vi "Initialise camera.vi"(8 "error in (no error) 2":errorcluster, 10 "Camera configuration":T4={"Temperature"=-70.0, "Exposure (sec)"=0.01, "EMGain"=3500.0, "ClearMode"=1.0, "ReadoutMode"=2.0, "ADC Gain"=-1} {"ADC Gain" items=["Use current ADC"=-1, "Use the fastest ADC"=-2, "Use the slowest ADC"=-3]; "ReadoutMode" items=["Normal readout"=1.0, "Frame transfer readout"=2.0, "MPP readout"=3.0, "Frame transfer MPP"=4.0, "Alternate timing for normal readout"=5.0, "Alternate timing for frame transfer"=6.0, "Alternate timing for MPP"=7.0, "Alternate timing for frame transfer MPP"=8.0, "Interline"=9.0]; "ClearMode" items=["Clear never"=1.0, "Clear pre-exposure"=2.0, "Clear pre-sequence"=3.0, "Clear post-sequence"=4.0, "Clear pre- and post-sequence"=5.0, "Clear pre-exposure and post-sequence"=6.0]; "EMGain" format="%.2f"; "Exposure (sec)" format="%.3f"; "Temperature" format="%.2f"}, 11 "Acqusition Info":T8={"Number of Images"=1000, "Image type"=6, "Acquire / Focus Flag"=1} {"Image type" items=["8 bit unsigned"=1, "16 bit unsigned"=2, "8 bit signed"=6, "16 bit signed"=7, "32 bit signed"=3, "32 bit floating"=4, "64 bit floating"=5, "32 bit unsigned"=8]}) -> (0 "error out":errorcluster, 2 "Camera Info":T6, 3 "Imafe Info":T5)   [LabVIEW 2012, in "DAQCascade512.lvclass"]
uses:
  DAQCascade512.lvclass
  OLD_apparatus_VI/VI/Image_type.ctl
  OLD_apparatus_VI/VI/Clearing_mode.ctl
  OLD_apparatus_VI/VI/Readout_mode.ctl
  OLD_apparatus_VI/VI/ADC_gain.ctl
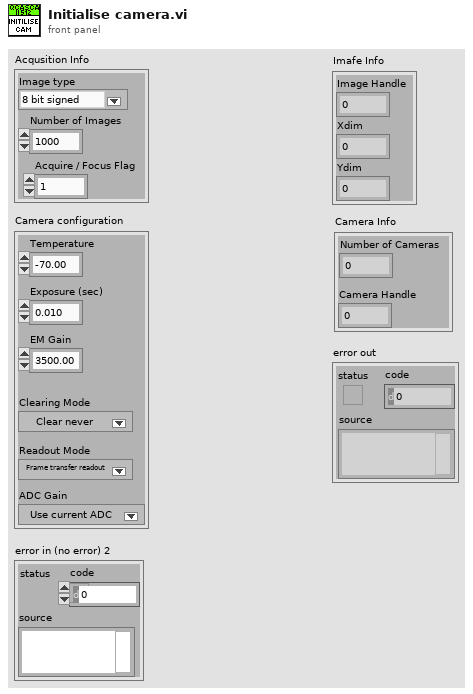
[diagram p1: front panel]
types:
  T1 = typedef "Clearing_mode.ctl" = dbl
  T2 = typedef "Readout_mode.ctl" = dbl
  T3 = typedef "ADC_gain.ctl" = i32
  T4 = cluster{"Temperature":dbl, "Exposure (sec)":dbl, "EMGain":dbl, "ClearMode":T1, "ReadoutMode":T2, "ADC Gain":T3}
  T5 = cluster{"Image Handle":u32, "Xdim":u32, "Ydim":u32}
  T6 = cluster{"Number of Cameras":i32, "Camera Handle":u32}
  T7 = typedef "Image_type.ctl" = u32
  T8 = cluster{"Number of Images":u32, "Image type":T7, "Acquire / Focus Flag":u32}
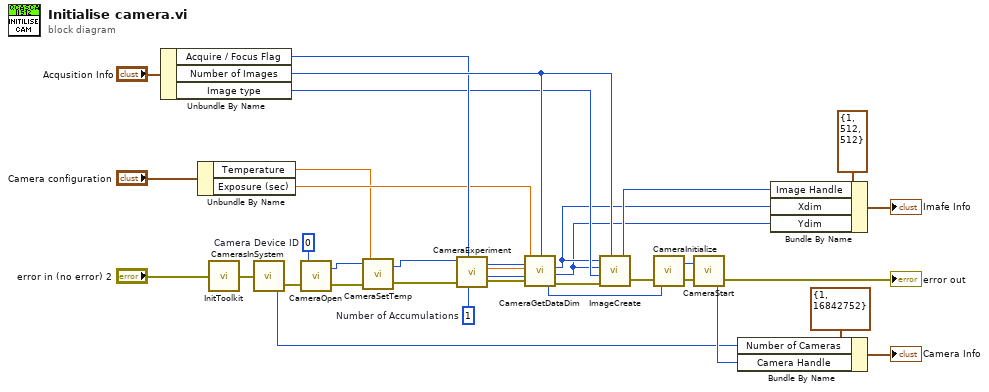
[diagram p0: block diagram]
diagram:
  w26 = u32 1  # Number of Accumulations
  w32 = u32 0  # Camera Device ID
  n1 = Unbundle By Name("Acqusition Info") -> ("Acquire / Focus Flag"=w13:u32, "Number of Images"=w14:u32, "Image type"=w12:T7)
  n2 = Unbundle By Name("Camera configuration") -> ("Temperature"=w10:dbl, "Exposure (sec)"=w11:dbl)
  n3 = call <userlib>:"InitToolkit.vi"("error in"="error in (no error) 2") -> ("error out"=w20:errorcluster)
  n4 = call <userlib>:"CamerasInSystem.vi"("error in"=w20) -> ("Number of Cameras"=w1:i32, "error out"=w27:errorcluster)
  n5 = call <userlib>:"CameraOpen.vi"("error in"=w27, "Camera Device ID"=w32) -> ("error out"=w30:errorcluster, "Camera Handle"=w31:u32)
  n6 = call <userlib>:"CameraSetTemp.vi"("error in (no error)"=w30, "Temperature"=w10, "Camera Handle"=w31) -> ("error out"=w19:errorcluster, "Camera Handle"=w18:u32)
  n7 = call <userlib>:"CameraExperiment.vi"("Number of Accumulations"=w26, "Acquire / Focus Flag"=w13, "error in"=w19, "Number of Images"=w14, "Exposure (sec)"=w11, "Camera Handle"=w18) -> ("error out"=w29:errorcluster, "Camera Handle"=w22:u32)
  n8 = call <userlib>:"CameraGetDataDim.vi"("Camera Handle"=w22, "error in"=w29) -> ("Camera Handle"=w21:u32, "Xdim"=w8:u32, "Ydim"=w7:u32, "error out"=w28:errorcluster)
  n9 = call <userlib>:"ImageCreate.vi"("X dimension"=w8, "Y dimension"=w7, "Data Type"=w12, "error in"=w28, "Number Of Frames"=w14) -> ("Image Handle"=w9:u32, "error out"=w24:errorcluster)
  n10 = call <userlib>:"CameraInitialize.vi"("error in"=w24, "Camera Handle"=w21) -> ("error out"=w23:errorcluster, "Camera Handle"=w25:u32)
  n11 = call <userlib>:"CameraStart.vi"("error in"=w23, "Camera Handle"=w25) -> ("error out"=→"error out":errorcluster, "Camera Handle"=w2:u32)
  n12 = Bundle By Name(cluster=T6 {"Number of Cameras"=1, "Camera Handle"=16842752} ("Camera Info"), "Number of Cameras"=w1, "Camera Handle"=w2) -> (→"Camera Info":T6)
  n13 = Bundle By Name(cluster=T5 {"Image Handle"=1, "Xdim"=512, "Ydim"=512} ("Imafe Info"), "Image Handle"=w9, "Xdim"=w8, "Ydim"=w7) -> (→"Imafe Info":T5)
